vi "Do.vi"(8 "error in (no error)":errorcluster, 10 "Actor in":refnum<class "Actor.lvclass">, 11 "Init Msg":refnum<class "Init Msg.lvclass">) -> (0 "error out":errorcluster, 2 "Actor out":refnum<class "Actor.lvclass">)   [LabVIEW 2023, in "ZWO_ASI.lvlib" / "Init Msg.lvclass"]
doc: "This VI delivers the message to the actor by calling the appropriate method(s) on the actor."
uses:
  Init Msg.lvclass
  9ef47adc-f318-494c-9b8b-6df3216d6863.vi
  ZWO_ASI/ZWO_ASI.lvclass
  <vilib>/ActorFramework/Actor/Actor.lvclass
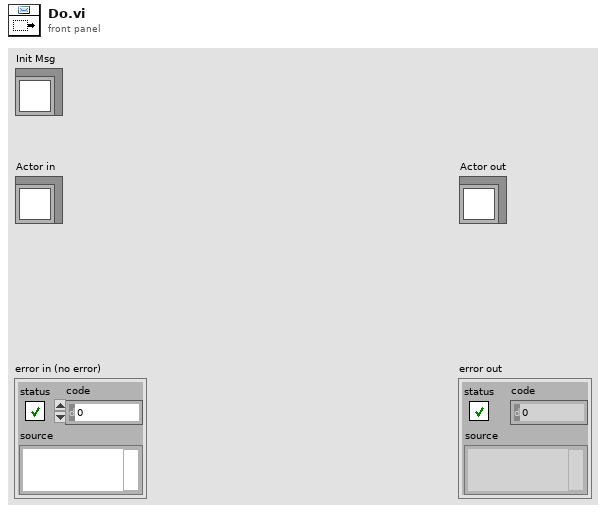
[diagram p1: front panel]
types:
  T1 = cluster{"address type":enum16{"VISA", "Index"}, "Address":string[]}
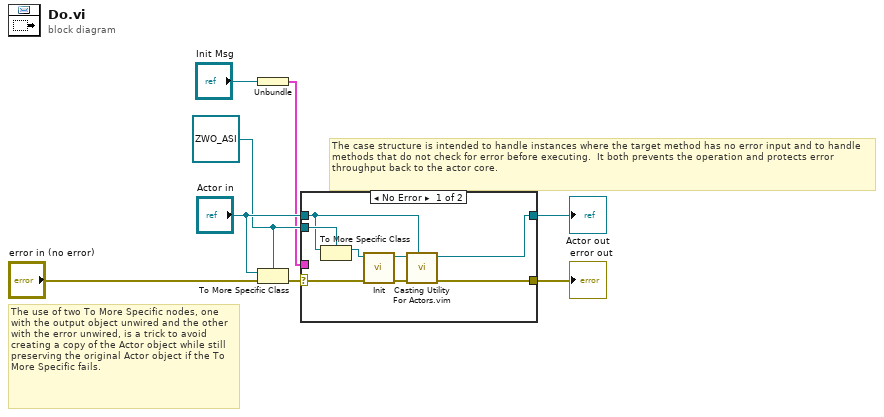
[diagram p0: block diagram]
diagram:
  w2 = refnum<class "ZWO_ASI.lvclass"> refnum ("Actor in")
  # "The use of two To More Specific nodes, one with the output object unwired and the other with the error unwired, is a trick to avoid creating a copy of the Actor object while still preserving the original Actor object if the To More Specific fails."
  # "The case structure is intended to handle instances where the target method has no error input and to handle methods that do not check for error before executing.  It both prevents the operation and protects error throughput back to the actor core."
  n1 = Unbundle("Init Msg") -> (w1:T1)
  n2 = To More Specific Class(target class=w2, reference="Actor in", error in="error in (no error)") -> (error out=w6:errorcluster)  [unwired: 1 out]
  n3 = case shown="No Error" w6 {
    selector: w6 -> [w16 w18]
    tunnel: [w10 w18] -> w5
    tunnel: [w11 w17] -> w4
    tunnel: "Actor in" -> [w13 w17]
    tunnel: w2 -> [w14 _]
    tunnel: w1 -> [_ _]
    frame No Error {
      n4 = To More Specific Class(target class=w14, reference=w13) -> (specific class reference=w15:refnum<class "ZWO_ASI.lvclass">)  [unwired: 1 in, 1 out]
      n5 = call-dynamic "Init.vi"("error in (no error)"=w16, "ZWO_ASI in"=w15) -> ("error out"=w9:errorcluster, "ZWO_ASI out"=w12:refnum<class "ZWO_ASI.lvclass">)  [unwired: 8 in]
      n6 = call "Casting Utility For Actors.vim"("type"=w13, "error in (no error)"=w9, "Actor in"=w12) -> ("error out"=w10:errorcluster, "Actor out"=w11:refnum<class "Actor.lvclass">)  [unwired: 7 in]
    }
    frame Error {
      # "If type check fails, pass the original object out again."
    }
  }
  "error out" <- w5
  "Actor out" <- w4
